vi "x_control_test.vi"() -> ()   [LabVIEW 2012]
uses:
  Key_Xcontrol.xctl
panel:
  out "KEY_Value Indicator":T1(ring) caption="KEY_Value"
  in  "KEY_Value Control":T1(ring) caption="KEY_Value"
  in  "沥瘤":bool
  out "Key_Indicator":u8(xcontrol)
  in  "Key_Xcontrol":u8(xcontrol)
  # "LED 甫 努腐窍咯 Key"
  # "LED 甫 喘矾焊技夸"
  # "KEY_Value 甫 函版秦 焊技夸"
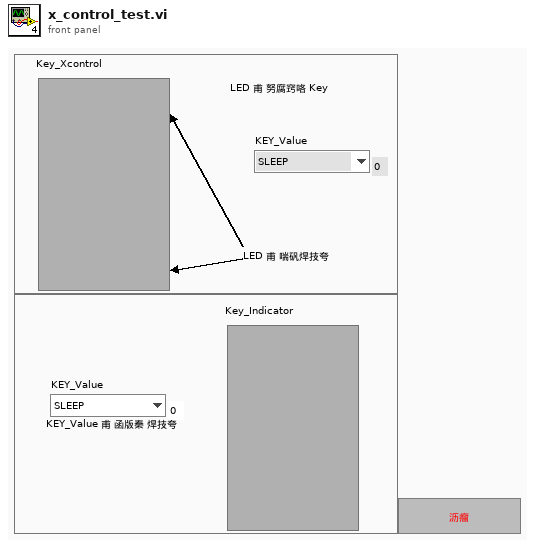
[diagram p1: front panel]
types:
  T1 = enum16{"SLEEP", "B+", "ACC", "IGN", "START", "IDLE"}
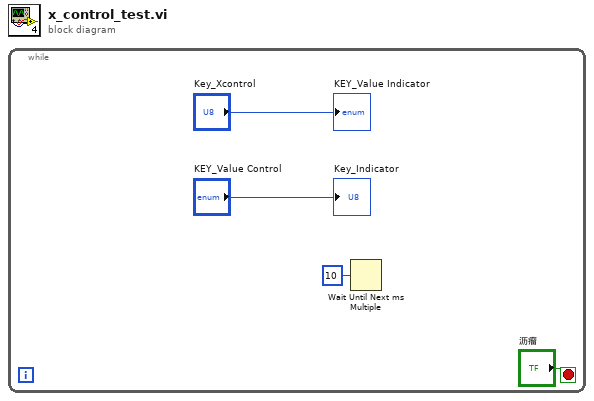
[diagram p0: block diagram]
diagram:
  n1 = while {
    stop <- "沥瘤" stop-if-true
    n2 = Wait Until Next ms Multiple(millisecond multiple=u32 10 ("ms 硅荐")) -> ()  [unwired: 1 out]
    "Key_Indicator" <- "KEY_Value Control"
    "KEY_Value Indicator" <- "Key_Xcontrol"
  }
